vi "temperat.vi"(4 "error in (no error)":errorcluster, 7 "VISA resource name":refnum<visa-resource-name>) -> (0 "error out":errorcluster, 1 "number":dbl, 2 "read buffer":string, 3 "VISA resource name out":refnum<visa-resource-name>)   [LabVIEW 2009]
uses:
  <vilib>/Instr/_visa.llb/VISA Configure Serial Port (Instr).vi
  <vilib>/Analysis/NI_AALBase.lvlib
panel:
  out "number 2":dbl
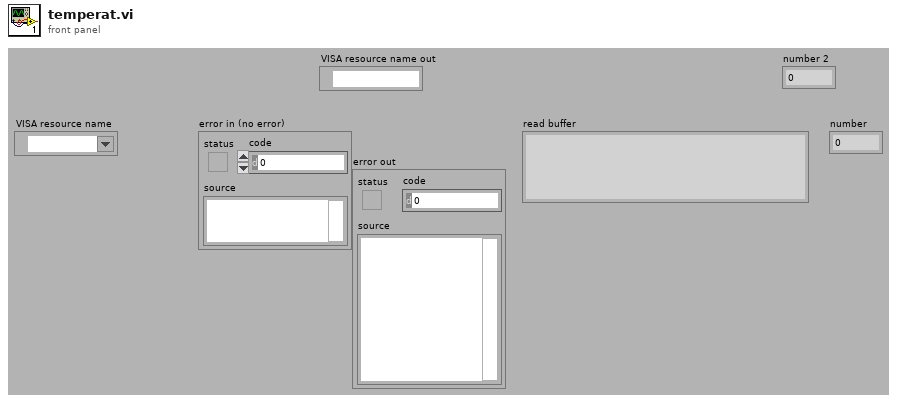
[diagram p1: front panel]
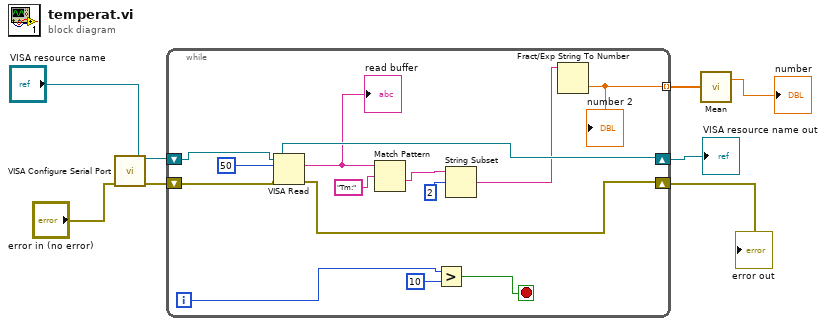
[diagram p0: block diagram]
diagram:
  n1 = call-poly "VISA Configure Serial Port"("VISA resource name"="VISA resource name", "error in (no error)"="error in (no error)") -> ("VISA resource name out"=w5:refnum<visa-resource-name>, "error out"=w8:errorcluster)  [unwired: 12 in]
  n2 = while {
    shift-right: [w21] -> w2
    shift-left: w5 -> [w11]
    shift-right: [w13] -> w1
    shift-left: w8 -> [w10]
    tunnel: [w19] -> w4 mode=indexing
    i -> [w9]
    stop <- w20 stop-if-true
    n3 = VISA Read(VISA resource name=w11, byte count=u32 50, error in (no error)=w10) -> (VISA resource name out=w21:refnum<visa-resource-name>, read buffer=w18:string, error out=w13:errorcluster)  [unwired: 1 out]
    "read buffer" <- w18
    n4 = Match Pattern(string=w18, regular expression="Tm:") -> (after substring=w15:string)  [unwired: 1 in, 3 out]
    n5 = Greater?(x=w9, y=u32 10) -> (0:w20:bool)
    n6 = String Subset(string=w15, offset (0)=2) -> (substring=w14:string)  [unwired: 1 in]
    n7 = Fract/Exp String To Number(string=w14) -> (number=w19:dbl)  [unwired: 3 in, 1 out]
    "number 2" <- w19
  }
  "VISA resource name out" <- w2
  "error out" <- w1
  n8 = call <vilib>:"Mean.vi"("X"=w4) -> ("mean"=→"number":dbl)  [unwired: 1 out]
